vi "Unload VI From Memory.vi"(8 "error in (no error)":errorcluster, 10 "VI Path":path, 11 "Session in":refnum<class "Session.lvclass">) -> (0 "error out":errorcluster, 3 "Session out":refnum<class "Session.lvclass">)   [LabVIEW 2020, in "Save for Previous Version.lvlib" / "Session.lvclass"]
uses:
  Session.lvclass
  Session.lvclass/Session.ctl
  <userlib>/_OpenG.lib/file/file.llb/Append Path to Root if Relative - Scalar__ogtk.vi
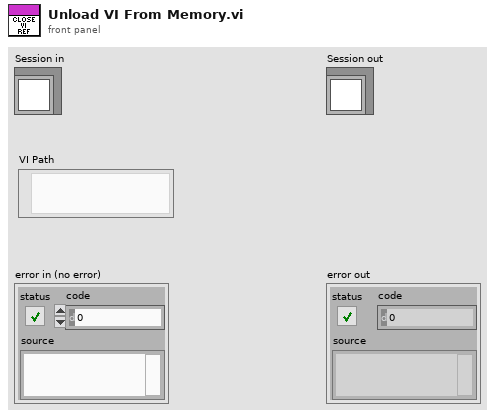
[diagram p1: front panel]
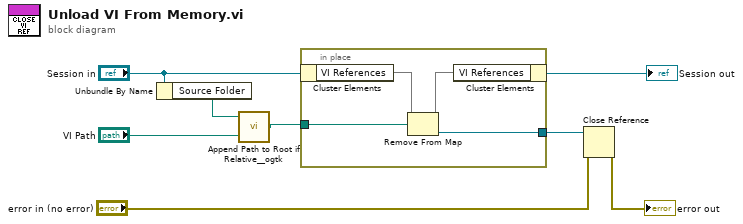
[diagram p0: block diagram]
diagram:
  n1 = Unbundle By Name("Session in") -> ("Source Folder"=w4:path)
  n2 = call-poly <userlib>:"Append Path to Root if Relative__ogtk.vi"("Absolute or Relative Path"="VI Path", "Root Path"=w4) -> ("Absolute or Appended Path"=w2:path)
  n3 = in-place {
    in-place-border: w2 -> [w11]
    in-place-border: [w9] -> w7
    n4 = in-place-cluster #1("Session in") -> ("VI References"=w12:map{path, refnum<vi>})
    n5 = Remove From Map(10:w11, 11:w12) -> (1:w9:refnum<vi>, 3:w10:map{path, refnum<vi>})  [unwired: 1 out]
    n6 = in-place-cluster #1("VI References"=w10) -> (→"Session out":refnum<class "Session.lvclass">)
  }
  n7 = Close Reference(reference=w7, error in (no error)="error in (no error)") -> (error out=→"error out":errorcluster)
